vi "CTE_Analysis_Suite_InputMaker_FormatStringLP.vi"(8 "ERROR":dbl, 9 "VALUE":dbl, 11 "NAME":string) -> (3 "Output":string)   [LabVIEW 2012]
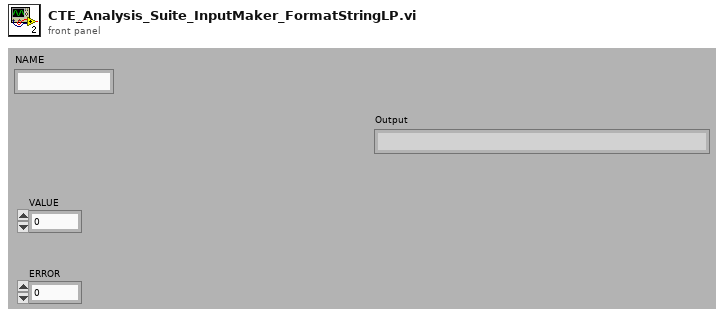
[diagram p1: front panel]
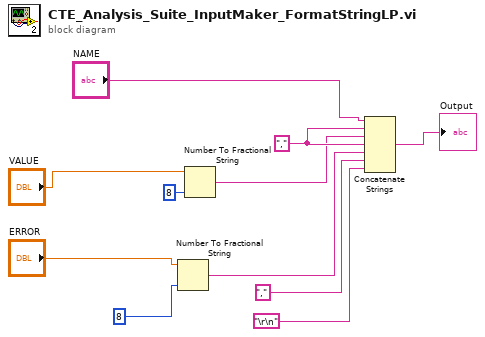
[diagram p0: block diagram]
diagram:
  w9 = ","
  n1 = Number To Fractional String(number="ERROR", precision (6)=i16 8) -> (F-format string=w5:string)  [unwired: 2 in]
  n2 = Number To Fractional String(number="VALUE", precision (6)=i16 8) -> (F-format string=w6:string)  [unwired: 2 in]
  n3 = Concatenate Strings("NAME", w9, w6, w9, w5, ",", "\r\n") -> (→"Output":string)
